vi "TAFTraceWindow_DeleteSubscriber.vi"(8 "ErrorIn":errorcluster, 10 "CmdData":variant, 11 "TAFTraceWindow in":refnum<class>) -> (0 "ErrorOut":errorcluster, 2 "ReplyData":variant, 3 "TAFTraceWindow out":refnum<class>, 4 "Exit":bool)   [LabVIEW 2021, in "TAFTraceWindow.lvclass"]
uses:
  TAFTraceWindow.lvclass
  TAFTraceWindow.lvclass/TAFTraceWindow.ctl
  4471e090-8e64-498f-a1be-083322230ba5.vi
  C:/Localdata/Projects/TriekselSoft/TriekselsoftApplicationFramework/Source/.Externals/Library_YAF/YAFTAF/YAFTAF.lvclass
  C:/Localdata/Projects/TriekselSoft/TriekselsoftApplicationFramework/Source/.Externals/Library_YAF/YActor/YActor.lvclass
  C:/Localdata/Projects/TriekselSoft/TriekselsoftApplicationFramework/Source/.Externals/Interface_UserInterface_IFrontPanel/IFrontPanel/IFrontPanel.lvclass
  C:/Localdata/Projects/TriekselSoft/TriekselsoftApplicationFramework/Source/IInterface/IInterface.lvclass
  C:/Localdata/Projects/TriekselSoft/TriekselsoftApplicationFramework/Source/.Externals/Interface_Object_ICreateDestroy/ICreateDestroy/ICreateDestroy.lvclass
  C:/Localdata/Projects/TriekselSoft/TriekselsoftApplicationFramework/Source/.Externals/Interface_Object_IPersistentData/IPersistentData/IPersistentData.lvclass
  C:/Localdata/Projects/TriekselSoft/TriekselsoftApplicationFramework/Source/.Externals/Interface_TAF_ITAFObject/ITAFObject/ITAFObject.lvclass
  C:/Localdata/Projects/TriekselSoft/TriekselsoftApplicationFramework/Source/.Externals/Library_TAF_TraceWindow/TAFTraceWindow/TAFTraceWindow.lvclass
  C:/Localdata/Projects/TriekselSoft/TriekselsoftApplicationFramework/Source/.Externals/INewOpenCVMat/INewOpenCVMat.lvclass
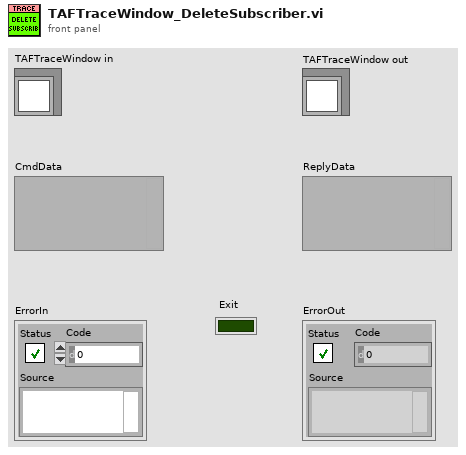
[diagram p1: front panel]
types:
  T1 = typedef "TAFTraceWindow.lvclass/FilterConfiguration.ctl" = cluster{"TraceColumn":i32, "FilterFunction":T2, "SearchText":string}
  T2 = typedef "TAFTraceWindow.lvclass/FilterFunction.ctl" = enum16{"Exact", "Regex"}
  T3 = cluster{"Name":string, "TargetQueue":refnum<queue>, "Configs":T1[]}[]
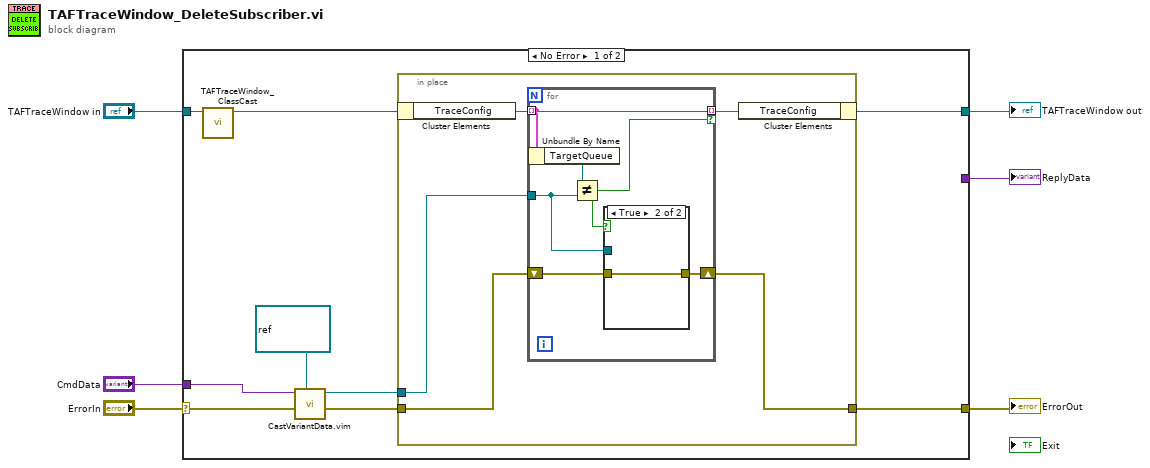
[diagram p0: block diagram]
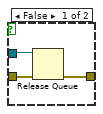
[diagram p2: hidden frame]
diagram:
  n1 = case shown="No Error" "ErrorIn" {
    selector: "ErrorIn" -> [w14 w32]
    tunnel: [w8 w32] -> w5
    tunnel: [_ w31] -> w3
    tunnel: "CmdData" -> [w12 w31]
    tunnel: "TAFTraceWindow in" -> [w13 w30]
    tunnel: [w11 w30] -> w1
    frame No Error {
      n2 = call "TAFTraceWindow_ClassCast.vi"("TAFTraceWindow in"=w13) -> ("TAFTraceWindow out"=w11:refnum<class "TAFTraceWindow.lvclass">)  [unwired: 10 in]
      n3 = call "CastVariantData.vim"("Type"=refnum<queue> refnum ("TraceQueue"), "ErrorIn"=w14, "DataIn"=w12) -> ("ErrorOut"=w9:errorcluster, "DataOut"=w10:refnum<queue>)  [unwired: 7 in]
      n4 = in-place {
        in-place-border: w10 -> [w18]
        in-place-border: w9 -> [w16]
        in-place-border: [w15] -> w8
        n5 = in-place-cluster #1(w11) -> ("TraceConfig"=w19:T3)
        n6 = for {
          tunnel: w19 -> [w24] mode=indexing
          tunnel: w18 -> [w22]
          tunnel: [w24] -> w17 mode=indexing if=w23
          shift-right: [w20] -> w15
          shift-left: w16 -> [w21]
          n7 = Unbundle By Name(w24) -> ("TargetQueue"=w25:refnum<queue>)
          n8 = Not Equal?(x=w25, y=w22) -> (x != y?=w23:bool)
          n9 = case shown="True" w23 {
            tunnel: w22 -> [w28 _]
            tunnel: w21 -> [w27 w29]
            tunnel: [w26 w29] -> w20
            frame False {
              n10 = Release Queue(queue=w28, error in (no error)=w27) -> (error out=w26:errorcluster)  [unwired: 1 in, 2 out]
            }
            frame True {
            }
          }
        }
        n11 = in-place-cluster #1("TraceConfig"=w17) -> ()  [unwired: 1 out]
      }
    }
    frame Error {
    }
  }
  "ErrorOut" <- w5
  "TAFTraceWindow out" <- w1
  "ReplyData" <- w3
